vi "贪吃蛇.vi"() -> ()   [LabVIEW 2013]
uses:
  <vilib>/Utility/inputDevices.llb/keyboardAcquire.vi
panel:
  out "分":dbl
  in  "速\n度":u16(slide)=280 min=100 max=500 step=100 scale=100.0..500.0
  in  "停止按钮":bool
  out "显示器":bool[][](array[boolean])
  # "贪吃蛇V1.0\n方向WSAD"
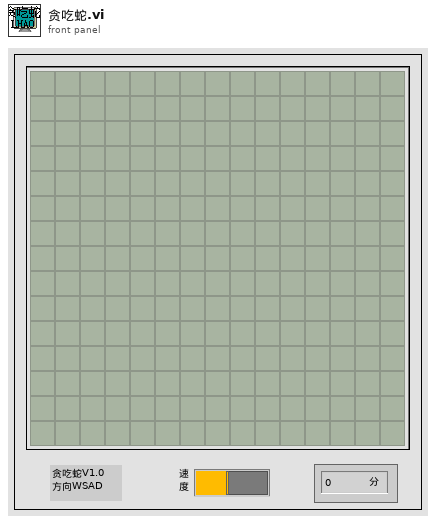
[diagram p1: front panel]
types:
  T1 = enum16{"0", "1", "2", "3", "4", "5", "6", "7", "8", "9", "A", "B", "C", "D", "E", "F", "G", "H", "I", "J", "K", "L", "M", "N", "O", "P", "Q", "R", "S", "T", "U", "V", "W", "X", "Y", "Z", "F1", "F2", "F3", "F4", "F5", "F6", "F7", "F8", "F9", "F10", "F11", "F12", "F13", "F14", "F15", "ADD", "BACK", "BACKSLASH", "CAPITAL", "COMMA", "DECIMAL", "DELETE", "DIVIDE", "DOWN", "END", "EQUALS", "ESCAPE", "GRAVE (`)", "HOME", "INSERT", "LBRACKET", "LCONTROL", "LEFT", "L ALT", "LSHIFT", "LWIN", "MINUS", "MULTIPLY", "NEXT", "NUMLOCK", "NUMPAD_0", "NUMPAD_1", "NUMPAD_2", "NUMPAD_3", "NUMPAD_4", "NUMPAD_5", "NUMPAD_6", "NUMPAD_7", "NUMPAD_8", "NUMPAD_9", "PAUSE", "PERIOD", "PRIOR (PG UP)", "RBRACKET", "RCONTROL", "RETURN", "RIGHT", "R ALT", "RSHIFT", "RWIN", "SCROLL", "SEMICOLON", "SLASH", "SPACE", "SUBTRACT", "TAB", "UP", "ENTER (num pad)", "' (quote)"}[]
  T2 = enum16{"0", "1", "2", "3", "4", "5", "6", "7", "8", "9", "A", "B", "C", "D", "E", "F", "G", "H", "I", "J", "K", "L", "M", "N", "O", "P", "Q", "R", "S", "T", "U", "V", "W", "X", "Y", "Z", "F1", "F2", "F3", "F4", "F5", "F6", "F7", "F8", "F9", "F10", "F11", "F12", "F13", "F14", "F15", "ADD", "BACK", "BACKSLASH", "CAPITAL", "COMMA", "DECIMAL", "DELETE", "DIVIDE", "DOWN", "END", "EQUALS", "ESCAPE", "GRAVE (`)", "HOME", "INSERT", "LBRACKET", "LCONTROL", "LEFT", "L ALT", "LSHIFT", "LWIN", "MINUS", "MULTIPLY", "NEXT", "NUMLOCK", "NUMPAD_0", "NUMPAD_1", "NUMPAD_2", "NUMPAD_3", "NUMPAD_4", "NUMPAD_5", "NUMPAD_6", "NUMPAD_7", "NUMPAD_8", "NUMPAD_9", "PAUSE", "PERIOD", "PRIOR (PG UP)", "RBRACKET", "RCONTROL", "RETURN", "RIGHT", "R ALT", "RSHIFT", "RWIN", "SCROLL", "SEMICOLON", "SLASH", "SPACE", "SUBTRACT", "TAB", "UP", "ENTER (num pad)", "' (quote)"}
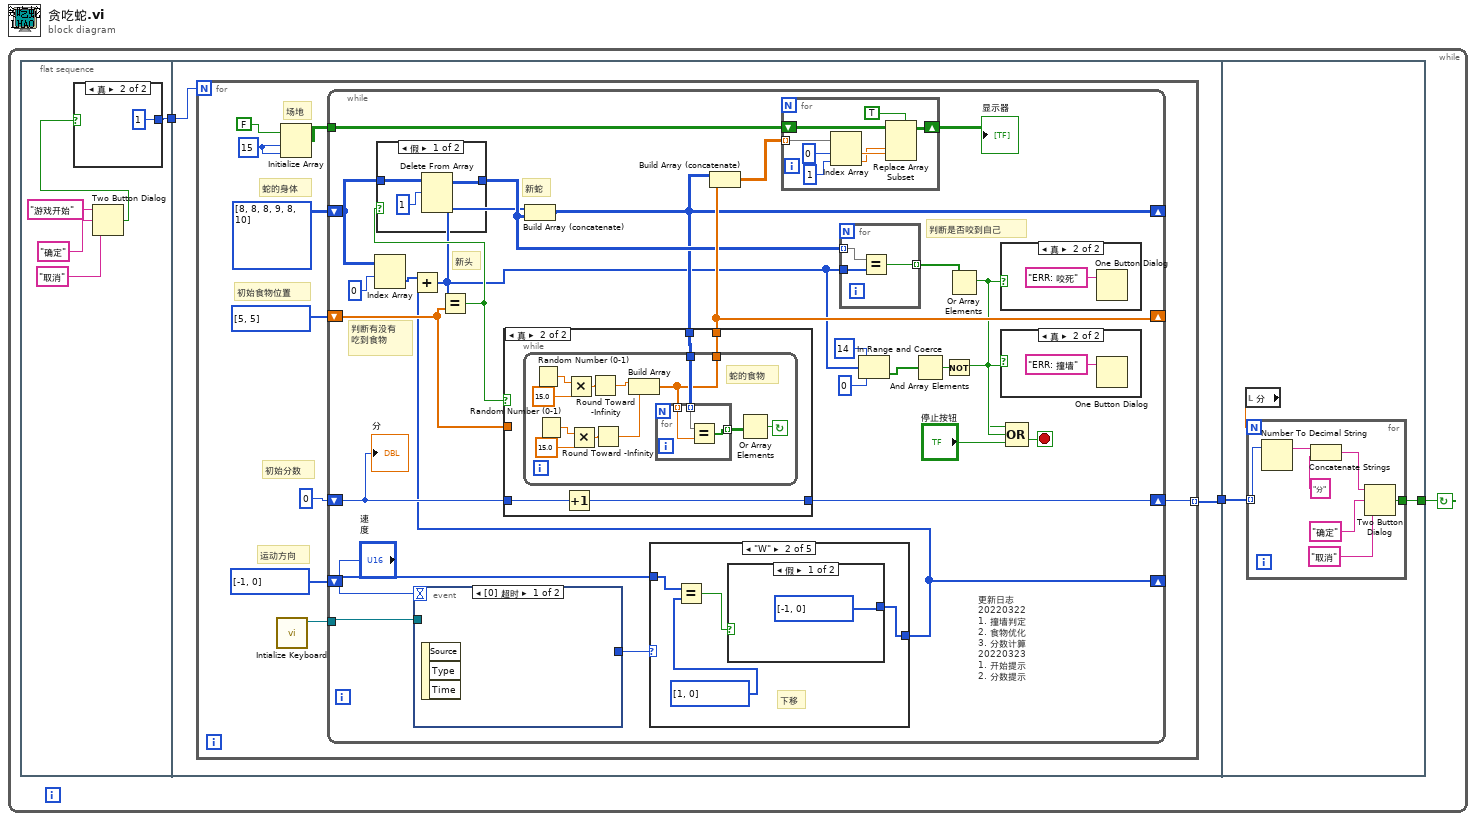
[diagram p0: block diagram]
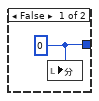
[diagram p2: hidden frame]
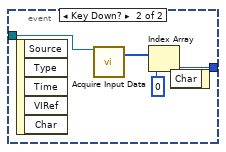
[diagram p7: hidden frame]
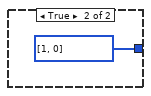
[diagram p9: hidden frame]
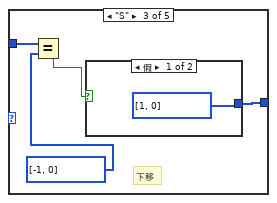
[diagram p10: hidden frame]
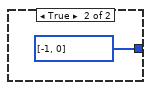
[diagram p11: hidden frame]
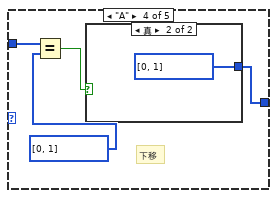
[diagram p12: hidden frame]
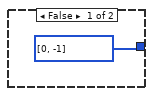
[diagram p13: hidden frame]
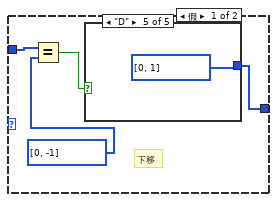
[diagram p14: hidden frame]
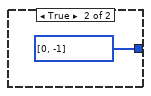
[diagram p15: hidden frame]
diagram:
  n1 = while {
    stop <- w1 continue-if-true
    n2 = flat-sequence {
      tunnel: [w6] -> w3
      tunnel: [w12] -> w2
      tunnel: w3 -> [w11]
      tunnel: w2 -> [w119]
      tunnel: [w118] -> w1
      frame #0 {
        n3 = Two Button Dialog(message="游戏开始" ("消息"), 1:"取消" ("F按钮名称（“取消”）"), 2:"确定" ("T按钮名称（“确定”）")) -> (T button?=w5:bool)
        n4 = case shown="真" w5 {
          tunnel: [w9 1] -> w6
          frame False {
            w9 = 0
            n5 = local write "分"(w9) -> ()
          }
          frame True {
          }
        }
      }
      frame #1 {
        n6 = for {
          N: w11 -> [_]
          tunnel: [w13] -> w12 mode=indexing
          w17 = 15 ("维数大小")
          # "初始分数"
          # "初始食物位置"
          # "场地"
          # "运动方向"
          # "蛇的身体"
          n7 = call <vilib>:"Intialize Keyboard.vi"() -> ("device ID"=w16:refnum<k1>)  [unwired: 10 in, 1 out]
          n8 = Initialize Array(FALSE, w17, w17) -> (w20:bool[][])
          n9 = while {
            tunnel: w20 -> [w49]
            shift-right: [w36] -> _
            shift-left: i32[][] [[8, 8], [8, 9], [8, 10]] -> [w43]
            tunnel: w16 -> [w45]
            shift-right: [w22] -> _
            shift-left: i32[] [-1, 0] -> [w46]
            shift-right: [w41] -> _
            shift-left: i32[] [5, 5] -> [w40]
            shift-right: [w27] -> w13
            shift-left: 0 -> [w24]
            stop <- w35 stop-if-true
            # "更新日志\n20220322\n1. 撞墙判定\n2. 食物优化\n3. 分数计算\n20220323\n1. 开始提示\n2. 分数提示"
            # "判断是否咬到自己"
            # "新蛇"
            # "新头"
            # "判断有没有\n吃到食物"
            n10 = Index Array(array=w43, index (row)=0 ("索引 (行)")) -> (element=w48:i32[])  [unwired: 1 in]
            n11 = event shown="[0] 超时" {
              selector: _ -> [_ _]
              dyn-events: _ -> [_ _]
              timeout: "速\n度" -> [_ _]
              tunnel: w45 -> [_ w81]
              tunnel: [_ w80] -> w44
              event Timeout {
                n12 = event-data() -> ()  [unwired: 1 in, 3 out]
              }
              event Key Down? {
                n13 = event-data() -> ()  [unwired: 1 in, 5 out]
                n14 = call-poly <vilib>:"Acquire Input Data.vi"("device ID"=w81) -> ("keys pressed"=w83:T1)  [unwired: 16 in, 2 out]
                n15 = Index Array(array=w83, index=0 ("索引")) -> (element=w80:T2)
                n16 = event-data() -> ()  [unwired: 2 in, 1 out]
              }
            }
            n17 = case shown="\"W\"" w44 {
              tunnel: w46 -> [w84 w88 w91 w98 w104]
              tunnel: [w84 w85 w92 w97 w103] -> w22
              frame "0", Default {
              }
              frame "W" {
                # "下移"
                n18 = Equal?(x=w88, y=i32[] [1, 0]) -> (x = y?=w86:bool)
                n19 = case shown="假" w86 {
                  tunnel: [i32[] [-1, 0] i32[] [1, 0]] -> w85
                  frame False {
                  }
                  frame True {
                  }
                }
              }
              frame "S" {
                # "下移"
                n20 = Equal?(x=w91, y=i32[] [-1, 0]) -> (x = y?=w93:bool)
                n21 = case shown="假" w93 {
                  tunnel: [i32[] [1, 0] i32[] [-1, 0]] -> w92
                  frame False {
                  }
                  frame True {
                  }
                }
              }
              frame "A" {
                # "下移"
                n22 = Equal?(x=w98, y=i32[] [0, 1]) -> (x = y?=w99:bool)
                n23 = case shown="真" w99 {
                  tunnel: [i32[] [0, -1] i32[] [0, 1]] -> w97
                  frame False {
                  }
                  frame True {
                  }
                }
              }
              frame "D" {
                # "下移"
                n24 = Equal?(x=w104, y=i32[] [0, -1]) -> (x = y?=w106:bool)
                n25 = case shown="假" w106 {
                  tunnel: [i32[] [0, 1] i32[] [0, -1]] -> w103
                  frame False {
                  }
                  frame True {
                  }
                }
              }
            }
            n26 = Add(x=w48, y=w22) -> (x+y=w31:i32[])
            n27 = Equal?(x=w31, y=w40) -> (x = y?=w39:bool)
            n28 = case shown="假" w39 {
              tunnel: w43 -> [w56 w58]
              tunnel: [w55 w58] -> w38
              frame False {
                n29 = Delete From Array(array=w56, length=1 ("长度")) -> (array with subset deleted=w55:i32[][])  [unwired: 2 in, 1 out]
              }
              frame True {
              }
            }
            n30 = Build Array (concatenate)(w31, w38) -> (w36:i32[][])
            n31 = case shown="真" w39 {
              tunnel: [w60 w64] -> w41
              tunnel: w40 -> [w60 _]
              tunnel: w36 -> [_ w63]
              tunnel: w24 -> [w59 w62]
              tunnel: [w59 w61] -> w27
              frame False {
              }
              frame True {
                n32 = while {
                  tunnel: [w67] -> w64
                  tunnel: w63 -> [w68]
                  stop <- w65 continue-if-true
                  # "蛇的食物"
                  n33 = Random Number (0-1)() -> (number: 0 to 1=w76:dbl)
                  n34 = Random Number (0-1)() -> (number: 0 to 1=w70:dbl)
                  n35 = Multiply(x=w76, y=15.0) -> (x*y=w75:dbl)
                  n36 = Multiply(x=w70, y=15.0) -> (x*y=w71:dbl)
                  n37 = Round Toward -Infinity(1:w75) -> (0:w73:dbl)
                  n38 = Round Toward -Infinity(1:w71) -> (0:w69:dbl)
                  n39 = Build Array(w73, w69) -> (w67:dbl[])
                  n40 = for {
                    tunnel: w68 -> [w79] mode=indexing
                    tunnel: w67 -> [w78] mode=indexing
                    tunnel: [w77] -> w66 mode=indexing
                    n41 = Equal?(x=w79, y=w78) -> (x = y?=w77:bool[])
                  }
                  n42 = Or Array Elements(Boolean array=w66) -> (logical OR=w65:bool)
                }
                n43 = Increment(x=w62) -> (x+1=w61:i32)
              }
            }
            n44 = Build Array (concatenate)(w36, w41) -> (w42:dbl[][])
            n45 = for {
              shift-right: [w109] -> w37
              shift-left: w49 -> [w113]
              tunnel: w42 -> [w114] mode=indexing
              n46 = Index Array(array=w114, index #1=0 ("索引"), index #2=1 ("索引")) -> (element #1=w112:dbl, element #2=w111:dbl)
              n47 = Replace Array Subset(array=w113, new element=TRUE, index (row)=w112, index (col)=w111) -> (w109:bool[][])
            }
            "显示器" <- w37
            n48 = for {
              tunnel: w38 -> [w53] mode=indexing
              tunnel: w31 -> [w54]
              tunnel: [w52] -> w23 mode=indexing
              n49 = Equal?(x=w53, y=w54) -> (x = y?=w52:bool)
            }
            n50 = In Range and Coerce(upper limit=14, x=w31, lower limit=0) -> (In Range?=w32:bool[])  [unwired: 1 out]
            n51 = And Array Elements(Boolean array=w32) -> (logical AND=w33:bool)
            n52 = Not(x=w33) -> (.not. x?=w28:bool)
            n53 = Or Array Elements(Boolean array=w23) -> (logical OR=w34:bool)
            n54 = case shown="真" w34 {
              frame False {
              }
              frame True {
                n55 = One Button Dialog(message="ERR: 咬死" ("消息")) -> ()  [unwired: 1 in, 1 out]
              }
            }
            n56 = case shown="真" w28 {
              frame False {
              }
              frame True {
                n57 = One Button Dialog(message="ERR: 撞墙" ("消息")) -> ()  [unwired: 1 in, 1 out]
              }
            }
            n58 = Compound Arithmetic op=OR(w28, w34, "停止按钮") -> (w35:bool)
            "分" <- w24
          }
        }
      }
      frame #2 {
        n59 = local read "分"() -> (w117:dbl)
        n60 = for {
          N: w117 -> [_]
          tunnel: w119 -> [w124] mode=indexing
          tunnel: [w120] -> w118
          n61 = Number To Decimal String(number=w124) -> (decimal integer string=w123:string)  [unwired: 1 in]
          n62 = Concatenate Strings(w123, "分" ("字符串")) -> (w121:string)
          n63 = Two Button Dialog(message=w121, 1:"取消" ("F按钮名称（“取消”）"), 2:"确定" ("T按钮名称（“确定”）")) -> (T button?=w120:bool)
        }
      }
    }
  }
